vi "Get Variables.vi"(8 "error in (no error)":errorcluster, 11 "Message Popup in":refnum<class "Arithmetic Operations.lvclass">) -> (0 "error out":errorcluster, 2 "Variables":variant, 3 "Message Popup out":refnum<class "Arithmetic Operations.lvclass">)   [LabVIEW 2016, in "Arithmetic Operations.lvclass"]
uses:
  Arithmetic Operations.lvclass
  Arithmetic Operations.lvclass/Arithmetic Operations.ctl
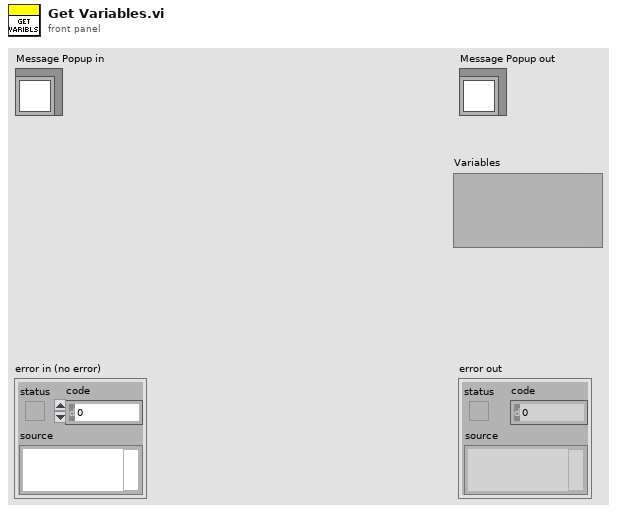
[diagram p1: front panel]
types:
  T1 = typedef "Arithmetic Operations.lvclass/Variables.ctl" = cluster{"Var1":dbl, "Var2":dbl}
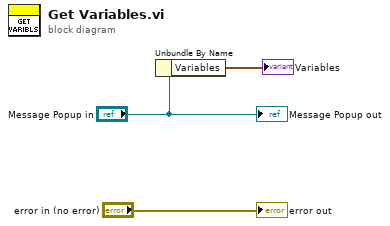
[diagram p0: block diagram]
diagram:
  n1 = Unbundle By Name("Message Popup in") -> ("Variables"=→"Variables":T1)
  "error out" <- "error in (no error)"
  "Message Popup out" <- "Message Popup in"
